vi "Aircraft Waypoints.vi"   [LabVIEW 2014]
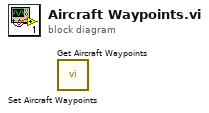
[diagram p0: block diagram]
diagram:
  n1 = call "Set Aircraft Waypoints.vi"() -> ()  [unwired: 11 in, 1 out]
  n2 = call "Get Aircraft Waypoints.vi"() -> ()  [unwired: 10 in, 2 out]
